vi "GetImageData.vi"(8 "error in (no error)":errorcluster, 11 "Picture in":refnum<class "Image.lvclass">) -> (0 "error out":errorcluster, 2 "image data":T1, 3 "Picture out":refnum<class "Image.lvclass">)   [LabVIEW 2021, in "Picture2D.lvlib" / "Image.lvclass"]
uses:
  Image.lvclass
  <vilib>/picture/picture.llb/imagedata.ctl
  Image.lvclass/Image.ctl
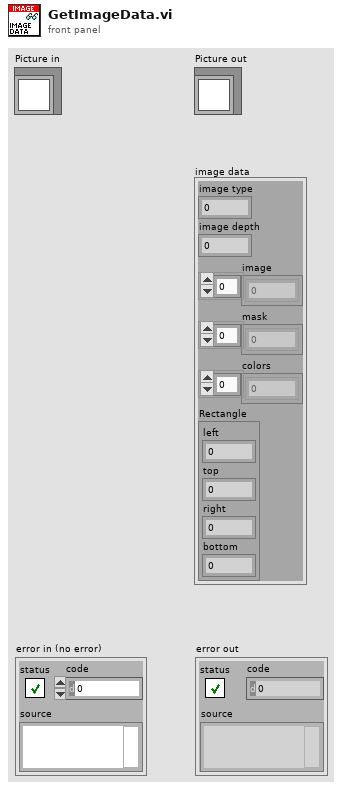
[diagram p1: front panel]
types:
  T1 = typedef "imagedata.ctl" = cluster{"image type":i32, "image depth":i32, "image":u8[], "mask":u8[], "colors":u32[], "Rectangle":cluster{"left":i16, "top":i16, "right":i16, "bottom":i16}}
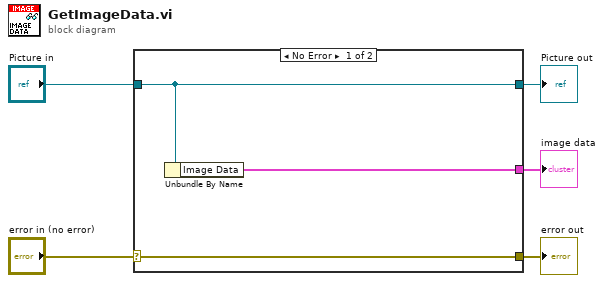
[diagram p0: block diagram]
diagram:
  n1 = case shown="No Error" "error in (no error)" {
    selector: "error in (no error)" -> [w8 w9]
    tunnel: [w8 w9] -> w4
    tunnel: [w7 w10] -> w2
    tunnel: "Picture in" -> [w7 w10]
    tunnel: [w6 _] -> w1
    frame No Error {
      n2 = Unbundle By Name(w7) -> ("Image Data"=w6:T1)
    }
    frame Error {
    }
  }
  "error out" <- w4
  "Picture out" <- w2
  "image data" <- w1
